vi "Get Next Point.vi"(0 "eye scan point iterator":refnum<class "niHighSpeedSerial N Point Eye Scan Point Iterator v1 Host.lvclass">, 11 "error in":errorcluster) -> (4 "eye scan point iterator out":refnum<class "niHighSpeedSerial N Point Eye Scan Point Iterator v1 Host.lvclass">, 6 "next point":T1, 15 "error out":errorcluster)   [LabVIEW 2014, in "niHighSpeedSerial N Point Eye Scan Point Iterator v1 Host.lvclass"]
doc: "Advances to the next point to be measured and returns its horizontal and vertical offset.\n\n<B>Input Parameters</B>\n\n<B>eye scan point iterator</B> is the incoming wire for the Eye Scan Point Iterator class object\n\n<B>error in</B> describes error conditions that occur before this node runs. This input provides standard 'error in' functionality.\n\n<B>Output Parameters</B>\n\n<B>eye scan point iterator out</B> is the outgoing wire for the Eye Scan Point Iterator class object\n\n<B>next point</B> is the next point to being measuring using Eye Scan\n\n<B>next point.horizontal offset</B> is the horizontal offset of the next point.\n\n<B>next point.vertical offset</B> is the vertical offset of the next point.\n\n<B>error out</B> contains error information. This output provides standard 'error out' functionality."
uses:
  <instrlib>/niHighSpeedSerial/Eye Scan/v1/Host/Impl/N Pt Iter/niHighSpeedSerial N Point Eye Scan Point Iterator v1 Host.lvclass
  <instrlib>/niHighSpeedSerial/Eye Scan/v1/Host/Common/Public/Point Offsets.ctl
  <instrlib>/niHighSpeedSerial/Eye Scan/v1/Host/Impl/N Pt Iter/niHighSpeedSerial N Point Eye Scan Point Iterator v1 Host.lvclass/niHighSpeedSerial N Point Eye Scan Point Iterator v1 Host.ctl
  <instrlib>/niHighSpeedSerial/Eye Scan/v1/Host/Common/niHighSpeedSerial Eye Scan Common v1 Host.lvlib
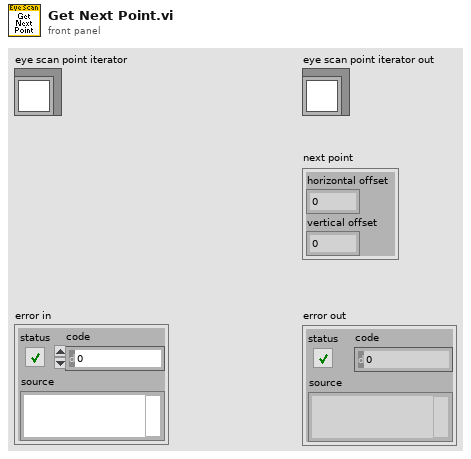
[diagram p1: front panel]
types:
  T1 = typedef "niHighSpeedSerial Eye Scan Common v1 Host.lvlib/Point Offsets.ctl" = cluster{"horizontal offset":i16, "vertical offset":i8}
  T2 = typedef "niHighSpeedSerial Eye Scan Common v1 Host.lvlib/Point.ctl" = cluster{"point offsets":T1, "sample count":u64, "error count":u64, "bit error rate":dbl}
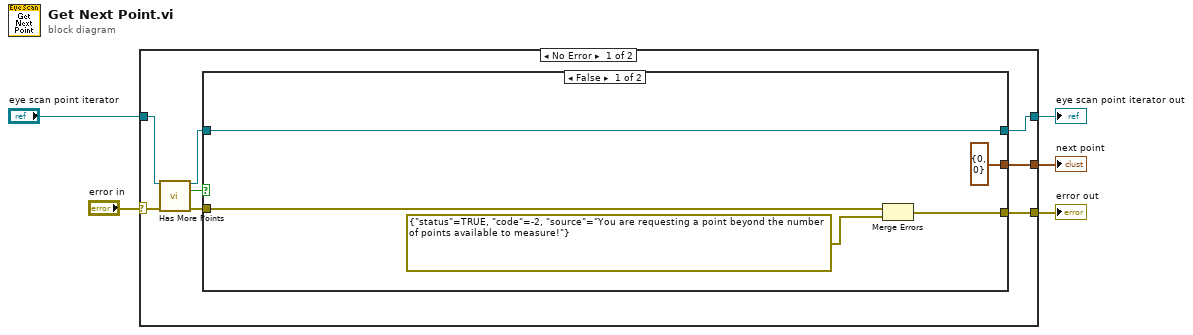
[diagram p0: block diagram]
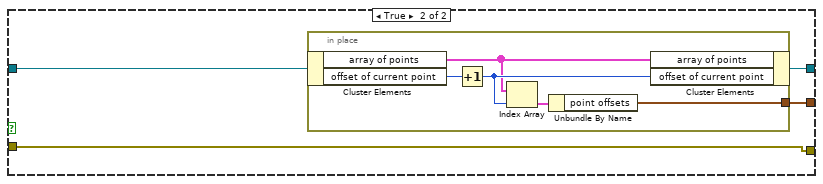
[diagram p2: hidden frame]
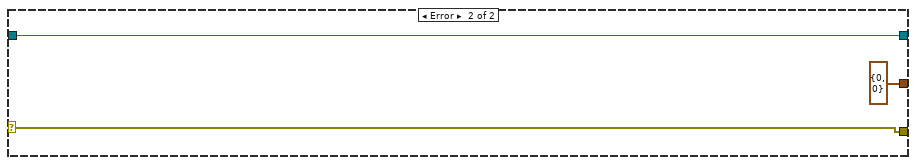
[diagram p3: hidden frame]
diagram:
  n1 = case shown="No Error" "error in" {
    selector: "error in" -> [w9 w30]
    tunnel: [w12 w30] -> w5
    tunnel: "eye scan point iterator" -> [w11 w29]
    tunnel: [w13 w29] -> w4
    tunnel: [w6 T1 {"horizontal offset"=0, "vertical offset"=0} ("Cluster")] -> w1
    frame No Error {
      n2 = call-dynamic "Has More Points.vi"("eye scan point iterator"=w11, "error in"=w9) -> ("eye scan point iterator out"=w10:refnum<class "niHighSpeedSerial N Point Eye Scan Point Iterator v1 Host.lvclass">, "has more points?"=w7:bool, "error out"=w8:errorcluster)  [unwired: 11 in]
      n3 = case shown="False" w7 {
        tunnel: [w15 w20] -> w13
        tunnel: [w16 w22] -> w12
        tunnel: w10 -> [w15 w21]
        tunnel: w8 -> [w18 w22]
        tunnel: [T1 {"horizontal offset"=0, "vertical offset"=0} ("Cluster") w19] -> w6
        frame False {
          n4 = Merge Errors(w18, errorcluster {"status"=TRUE, "code"=-2, "source"="You are requesting a point beyond the number of points available to measure!"} ("error out")) -> (w16:errorcluster)
        }
        frame True {
          n5 = in-place {
            in-place-border: [w23] -> w19
            n6 = in-place-cluster #1(w21) -> ("array of points"=w25:T2[], "offset of current point"=w27:i32)
            n7 = Increment(x=w27) -> (x+1=w26:i32)
            n8 = Index Array(array=w25, index=w26) -> (element=w24:T2)
            n9 = Unbundle By Name(w24) -> ("point offsets"=w23:T1)
            n10 = in-place-cluster #1("array of points"=w25, "offset of current point"=w26) -> (w20:refnum<class "niHighSpeedSerial N Point Eye Scan Point Iterator v1 Host.lvclass">)
          }
        }
      }
    }
    frame Error {
    }
  }
  "eye scan point iterator out" <- w4
  "error out" <- w5
  "next point" <- w1
